vi "InitApplication.vi"(8 "error in (no error)":errorcluster, 10 "Application Data in":T2, 11 "GUI Refs":T1) -> (0 "error out":errorcluster)   [LabVIEW 2019]
uses:
  Typedefs/#cluster_ApplicationData.ctl
  Typedefs/Acquisition Thread/#cluster_AcqQueueData.ctl
  Typedefs/Acquisition Thread/#enum_AcquisitionTask.ctl
  Typedefs/Saving Thread/#cluster_SavingQueueData.ctl
  Typedefs/Saving Thread/#enum_SavingTask.ctl
  Typedefs/#cluster_GUIRefs.ctl
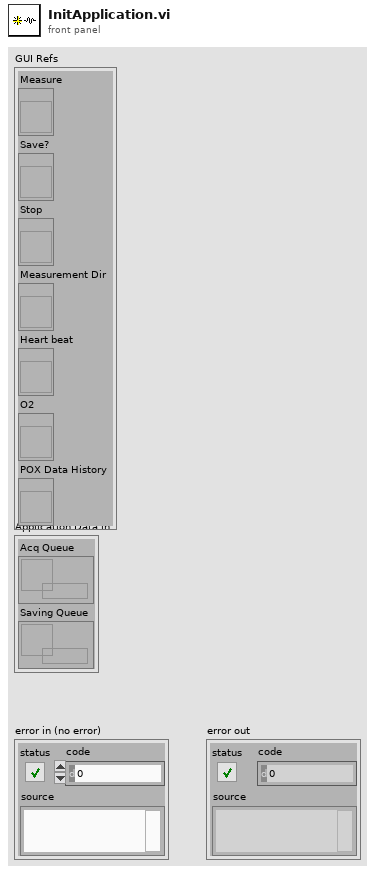
[diagram p1: front panel]
types:
  T1 = typedef "#cluster_GUIRefs.ctl" = cluster{"Measure":refnum<vi>, "Save?":refnum<vi>, "Stop":refnum<vi>, "Measurement Dir":refnum<vi>, "Heart beat":refnum<vi>, "O2":refnum<vi>, "POX Data History":refnum<vi>}
  T2 = typedef "#cluster_ApplicationData.ctl" = cluster{"Acq Queue":refnum<queue>, "Saving Queue":refnum<queue>}
  T3 = typedef "#cluster_AcqQueueData.ctl" = cluster{"Task":T4, "Data":variant}
  T4 = typedef "#enum_AcquisitionTask.ctl" = enum16{"Init", "Start", "Finish", "Close"}
  T5 = typedef "#cluster_AppConfiguration.ctl" = cluster{"Measurements Directory":path}
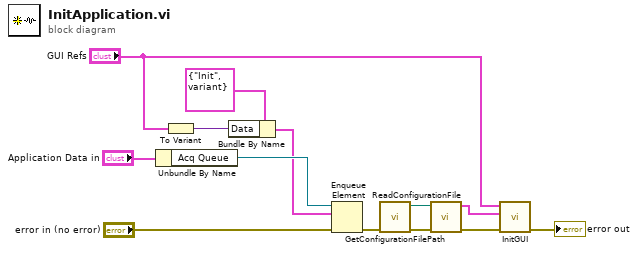
[diagram p0: block diagram]
diagram:
  n1 = Unbundle By Name("Application Data in") -> ("Acq Queue"=w7:refnum<queue>)
  n2 = To Variant(anything="GUI Refs") -> (Variant=w9:variant)
  n3 = Bundle By Name(cluster=T3 {"Task"=enum."Init", "Data"=variant} ("Acq Data"), "Data"=w9) -> (w6:T3)
  n4 = Enqueue Element(queue=w7, element=w6, error in (no error)="error in (no error)") -> (error out=w3:errorcluster)  [unwired: 1 in, 2 out]
  n5 = call "GetConfigurationFilePath.vi"() -> ("Configuration File Path"=w5:path)  [unwired: 11 in]
  n6 = call "ReadConfigurationFile.vi"("Error in"=w3, "Configuration File Path"=w5) -> ("Error out"=w2:errorcluster, "App Configuration"=w4:T5)  [unwired: 8 in]
  n7 = call "InitGUI.vi"("error in (no error)"=w2, "App Configuration"=w4, "GUI Refs"="GUI Refs") -> ("error out"=→"error out":errorcluster)  [unwired: 8 in]
